vi "usrp set tx freq.vi"(6 "tune_result":T1, 8 "error in (no error)":errorcluster, 9 "chan":u64, 10 "tune_request":T2={"target_freq"=0.0, "rf_freq_policy"=78, "@dummy control@"=0, "@dummy control@"=0, "@dummy control@"=0, "@dummy control@"=0, "rf_freq"=0.0, "dsp_freq_policy"=78, "@dummy control@"=0, "@dummy control@"=0, "@dummy control@"=0, "@dummy control@"=0, "dsp_freq"=0.0, "args"=0} {"rf_freq_policy" items=["UHD_TUNE_REQUEST_POLICY_NONE"=78, "UHD_TUNE_REQUEST_POLICY_AUTO"=65, "UHD_TUNE_REQUEST_POLICY_MANUAL"=77]; "dsp_freq_policy" items=["UHD_TUNE_REQUEST_POLICY_NONE"=78, "UHD_TUNE_REQUEST_POLICY_AUTO"=65, "UHD_TUNE_REQUEST_POLICY_MANUAL"=77]}, 11 "h":u64) -> (0 "error out":errorcluster, 1 "function return":u32(ring), 2 "tune_request out":T2={"target_freq"=0.0, "rf_freq_policy"=78, "@dummy control@"=0, "@dummy control@"=0, "@dummy control@"=0, "@dummy control@"=0, "rf_freq"=0.0, "dsp_freq_policy"=78, "@dummy control@"=0, "@dummy control@"=0, "@dummy control@"=0, "@dummy control@"=0, "dsp_freq"=0.0, "args"=0} {"rf_freq_policy" items=["UHD_TUNE_REQUEST_POLICY_NONE"=78, "UHD_TUNE_REQUEST_POLICY_AUTO"=65, "UHD_TUNE_REQUEST_POLICY_MANUAL"=77]; "dsp_freq_policy" items=["UHD_TUNE_REQUEST_POLICY_NONE"=78, "UHD_TUNE_REQUEST_POLICY_AUTO"=65, "UHD_TUNE_REQUEST_POLICY_MANUAL"=77]}, 3 "h 2":u64, 4 "tune_result out":T1, 5 "args":string)   [LabVIEW 2024, in "uhd.lvlib"]
doc: "UHD_API uhd_error uhd_usrp_set_tx_freq(uhd_usrp_handle h,\n uhd_tune_request_t* tune_request,\n size_t chan,\n uhd_tune_result_t* tune_result);"
uses:
  uhd.lvlib
  <vilib>/Utility/importsl/GetValueByPointer/datatype.ctl
  <vilib>/Utility/importsl/GetValueByPointer/GetValueByPointer.xnode
  uhd.so
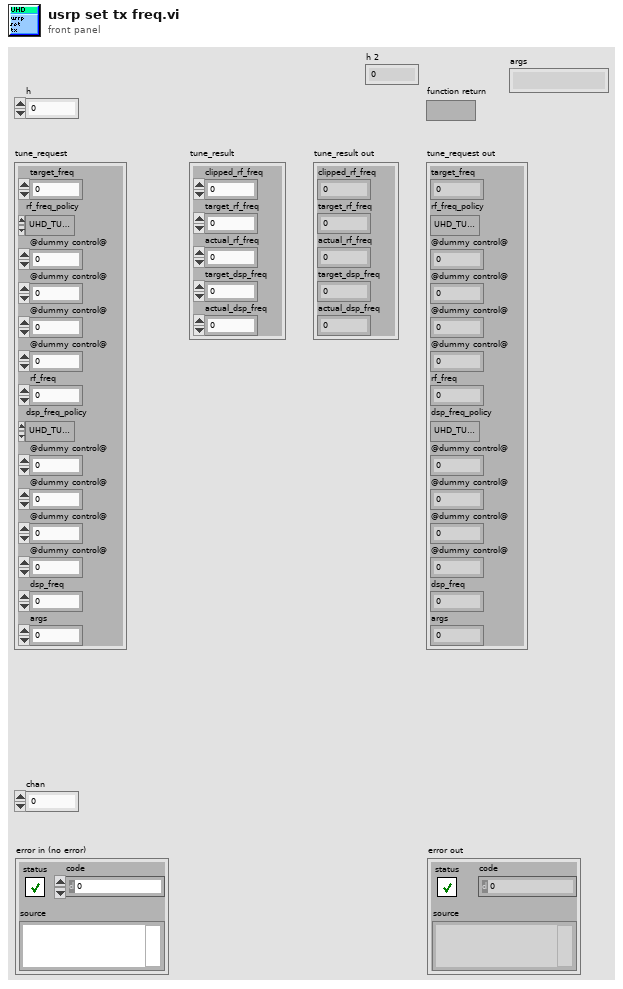
[diagram p1: front panel]
types:
  T1 = cluster{"clipped_rf_freq":dbl, "target_rf_freq":dbl, "actual_rf_freq":dbl, "target_dsp_freq":dbl, "actual_dsp_freq":dbl}
  T2 = cluster{"target_freq":dbl, "rf_freq_policy":u32, "@dummy control@":i8, "@dummy control@":i8, "@dummy control@":i8, "@dummy control@":i8, "rf_freq":dbl, "dsp_freq_policy":u32, "@dummy control@":i8, "@dummy control@":i8, "@dummy control@":i8, "@dummy control@":i8, "dsp_freq":dbl, "args":u64}
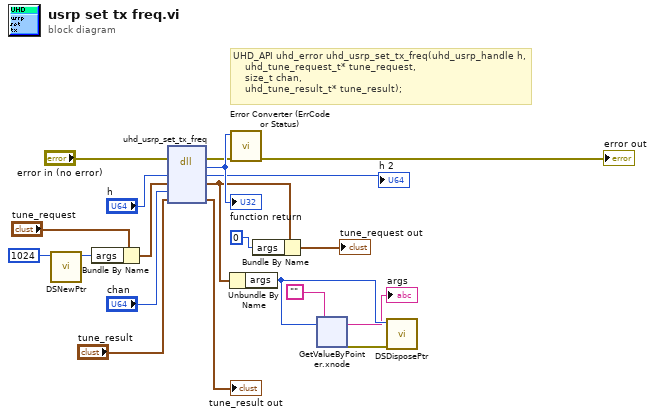
[diagram p0: block diagram]
diagram:
  # "UHD_API uhd_error uhd_usrp_set_tx_freq(uhd_usrp_handle h,\n    uhd_tune_request_t* tune_request,\n    size_t chan,\n    uhd_tune_result_t* tune_result);"
  n1 = call <vilib>:"DSNewPtr.vi"("Size"=u64 1024) -> ("Pointer"=w16:u64)  [unwired: 9 in, 1 out]
  n2 = Bundle By Name(cluster="tune_request", "args"=w16) -> (w15:T2)
  n3 = dll-call lib="uhd.*" fn="uhd_usrp_set_tx_freq"(error in="error in (no error)", "h"="h", "tune_request"=w15, "chan"="chan", "tune_result"="tune_result") -> (error out=w3:errorcluster, w20:u32, "h"=→"h 2":u64, "tune_request"=w10:T2, "tune_result"=→"tune_result out":T1)  [unwired: 3 in, 1 out]
  "function return" <- w20
  n4 = Unbundle By Name(w10) -> ("args"=w13:u64)
  n5 = call "Error Converter (ErrCode or Status).vi"("error in (no error)"=w3, "error code"=w20) -> ("error out"=→"error out":errorcluster)  [unwired: 9 in]
  n6 = Bundle By Name(cluster=w10, "args"=u64 0) -> (→"tune_request out":T2)
  n7 = xnode "GetValueByPointer.xnode"("Pointer"=w13, "InputType"="") -> ("Output"=→"args":string, "ErrorOut"=w14:errorcluster)  [unwired: 2 in]
  n8 = call <vilib>:"DSDisposePtr.vi"("error in (no error)"=w14, "Pointer"=w13) -> ()  [unwired: 9 in, 1 out]
